vi "Create.vi"(7 "VolatusAPI":refnum<class "VolatusAPI.lvclass">, 8 "error in (no error)":refnum<class "MultiErrors.lvclass">, 9 "Sequencer":refnum<class "MessageQ.lvclass">, 10 "Sequence Config":refnum<class "Sequence Config.lvclass">) -> (0 "error out":refnum<class "MultiErrors.lvclass">, 3 "Sequence out":refnum<class "Sequence.lvclass">)   [LabVIEW 2023, in "VolatusSeq.lvlib" / "Sequence.lvclass"]
uses:
  Sequence.lvclass
  VolatusErrorUtilities/MultiErrors/MultiErrors.lvclass
  VolatusSeqConfig/Sequence Config/Sequence Config.lvclass
  Volatus/VolatusAPI/VolatusAPI.lvclass
  Volatus/MessageQ/MessageQ.lvclass
  Sequence.lvclass/Sequence.ctl
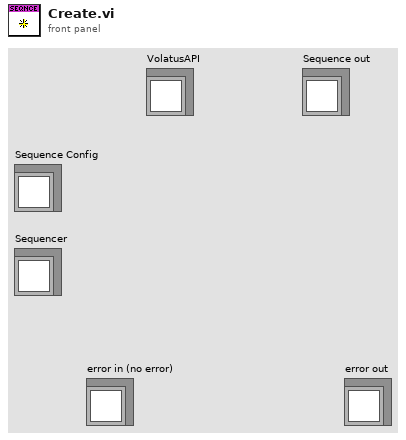
[diagram p1: front panel]
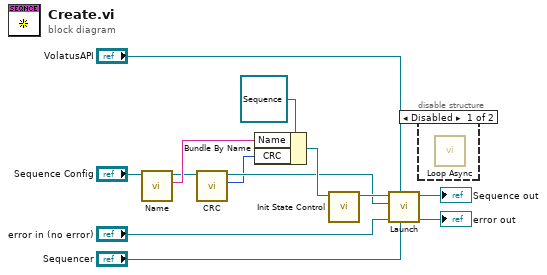
[diagram p0: block diagram]
diagram:
  n1 = call "Name.vi"("Sequence Config in"="Sequence Config") -> ("Name"=w11:string, "Sequence Config out"=w9:refnum<class "Sequence Config.lvclass">)  [unwired: 8 in, 1 out]
  n2 = call "CRC.vi"("Sequence Config in"=w9) -> ("CRC"=w2:u32, "Sequence Config out"=w3:refnum<class "Sequence Config.lvclass">)  [unwired: 9 in]
  n3 = Bundle By Name(cluster=refnum<class "Sequence.lvclass"> refnum ("Sequence in"), "Name"=w11, "CRC"=w2) -> (w6:refnum<class "Sequence.lvclass">)
  n4 = call "Init State Control.vi"("Sequence in"=w6) -> ("Sequence out"=w5:refnum<class "Sequence.lvclass">)  [unwired: 9 in, 1 out]
  n5 = call "Launch.vi"("Sequencer"="Sequencer", "VolatusAPI"="VolatusAPI", "error in (no error)"="error in (no error)", "Sequence Config"=w3, "Sequence in"=w5) -> ("error out"=→"error out":refnum<class "MultiErrors.lvclass">, "Sequence out"=→"Sequence out":refnum<class "Sequence.lvclass">)  [unwired: 5 in]
  n6 = disable-structure shown="Disabled" {
    frame Disabled {
      n7 = call "Loop Async.vi"() -> ()  [unwired: 12 in]
    }
    frame Enabled {
    }
  }
